vi "Get .ecc Type.vi"(8 "error in (no error)":errorcluster, 11 "Potentiostat Galvanostat in":refnum<class "Potentiostat Galvanostat.lvclass">) -> (0 "error out":errorcluster, 1 "Ecc Type":string, 2 "Ecc Type":enum16{"ecc", "ecc4"}(ring), 3 "Potentiostat Galvanostat out":refnum<class "Potentiostat Galvanostat.lvclass">)   [LabVIEW 2018, in "Potentiostat Galvanostat.lvclass"]
uses:
  Potentiostat Galvanostat.lvclass
  Potentiostat Galvanostat.lvclass/Potentiostat Galvanostat.ctl
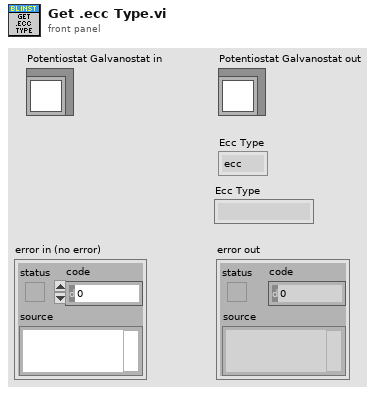
[diagram p1: front panel]
types:
  T1 = typedef "Potentiostat Galvanostat.lvclass/Device Code.ctl" = i32
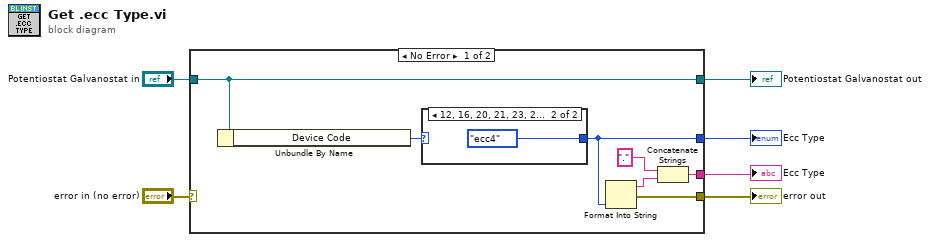
[diagram p0: block diagram]
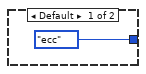
[diagram p2: hidden frame]
diagram:
  n1 = case shown="No Error" "error in (no error)" {
    selector: "error in (no error)" -> [_ w17]
    tunnel: [w8 w17] -> w1
    tunnel: [w13 w16] -> w4
    tunnel: "Potentiostat Galvanostat in" -> [w13 w16]
    tunnel: [w9 _] -> w3
    tunnel: [w10 _] -> w2
    frame No Error {
      n2 = Unbundle By Name(w13) -> ("Device Code"=w12:T1)
      n3 = case shown="12, 16, 20, 21, 23, 27, 32" w12 {
        tunnel: [enum16{"ecc", "ecc4"}."ecc" enum16{"ecc", "ecc4"}."ecc4"] -> w9
        frame Default {
        }
        frame 12, 16, 20, 21, 23, 27, 32 {
        }
      }
      n4 = Format Into String(w9) -> (resulting string=w7:string, error out=w8:errorcluster)  [unwired: 3 in]
      n5 = Concatenate Strings("." ("string"), w7) -> (w10:string)
    }
    frame Error {
    }
  }
  "error out" <- w1
  "Potentiostat Galvanostat out" <- w4
  "Ecc Type" <- w3
  "Ecc Type" <- w2
